vi "Waves.vi"(2 "Camera Queue":refnum<queue>, 3 "Wave Queue":refnum<queue>) -> (0 "error IO":errorcluster)   [LabVIEW 2016]
uses:
  controls/ModeEnum.ctl
  controls/Microscope Settings.ctl
  controls/ColourCalibration.ctl
  controls/CameraControlTypeDef.ctl
  controls/Hardware.ctl
  controls/PinOut.ctl
  <vilib>/Waveform/WDTOps.llb/WDT Waveform Duration DBL.vi
  <vilib>/DAQmx/create/channels.llb/DAQmx Create Channel (DO-Digital Output).vi
  <vilib>/DAQmx/create/channels.llb/DAQmx Create Channel (AO-Voltage-Basic).vi
panel:
  out "Duration":string
  out "Mixed Signal Graph 2":cluster{waveform(dbl)[], digitalwaveform[]}(graph)
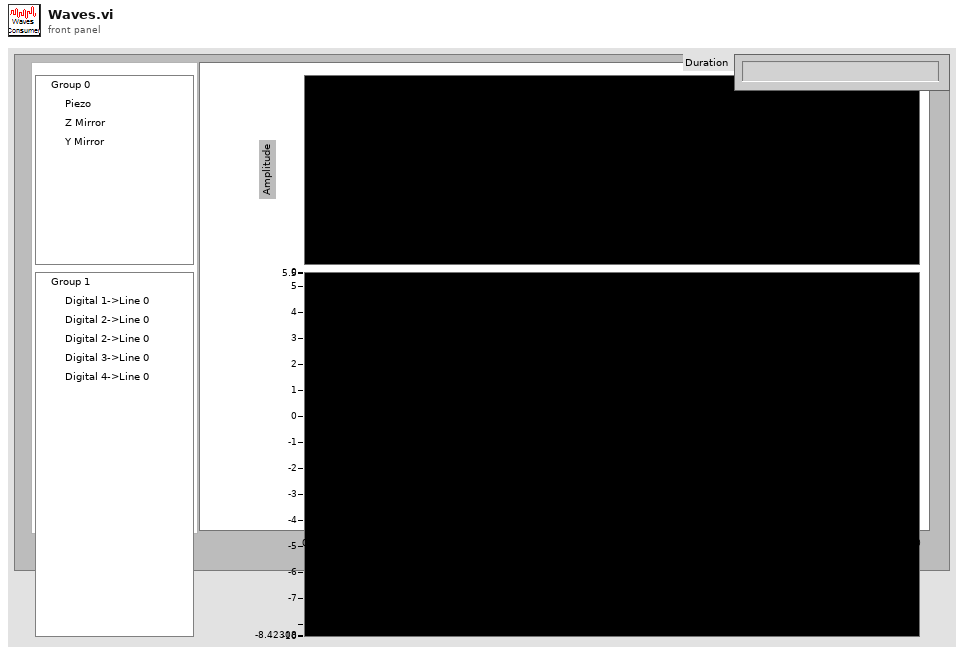
[diagram p1: front panel]
types:
  T1 = typedef "Microscope Settings.ctl" = cluster{"Mode":enum16{"Brightfield", "X", "XY", "XYZ", "XYZT", "XYZC", "Tweezers", "Virus"}, "Slit":cluster{"Scanning Mode":dbl, "Slit Width /%":dbl}, "Colour":T2, "Exposure/ms":dbl, "Piezo Position /um":dbl, "ROI":cluster{"X":cluster{"Start /px":dbl, "Step /px":dbl, "Range /px":dbl}, "Y":cluster{"Start /px":dbl, "Step /px":dbl, "Range /px":dbl}, "Z ":cluster{"Start /um":dbl, "Step/um":dbl, "Range /um":dbl}, "T ":cluster{"Start /s":dbl, "Step /s":dbl, "Range /s":dbl}}, "Samples per millisecond":dbl, "Relax/ms":dbl, "Readout Direction":dbl, "Trigger Source":dbl, "Camera Delay /ms":dbl, "Under Scan /ms":dbl, "Waveforms":cluster{"Analogue Out":waveform(dbl)[], "Digital Out":digitalwaveform[]}}
  T2 = typedef "ColourCalibration.ctl" = cluster{"Colour":cluster{"Laser":enum16{"Brightfield", "445", "488", "561", "647"}, "Filter":u16}, "Calibration Coordinates":cluster{"Top Left":dbl[], "Top Right":dbl[], "Bottom Left":dbl[], "Bottom Right":dbl[]}}[]
  T3 = typedef "Hardware.ctl" = enum16{"Stop", "RunCont", "EndCont", "Idle", "Update", "Run Waves"}
  T4 = typedef "ModeEnum.ctl" = enum16{"Idle", "Init", "generateWaves", "runWaves", "runWavesCont", "endWavesCont", "stop"}
  T5 = typedef "Microscope Settings.ctl" = cluster{"Mode":enum16{"Brightfield", "X", "XY", "XYZ", "XYZT", "XYZC", "Tweezers", "Virus"}, "Slit":cluster{"Scanning Mode":dbl, "Slit Width /%":dbl}, "Colour":cluster{"Laser":enum16{"Brightfield", "445", "488", "561", "647"}, "Filter":u16}[], "Exposure/ms":dbl, "Piezo Position /um":dbl, "ROI":cluster{"X":cluster{"Start /px":dbl, "Step /px":dbl, "Range /px":dbl}, "Y":cluster{"Start /px":dbl, "Step /px":dbl, "Range /px":dbl}, "Z ":cluster{"Start /um":dbl, "Step/um":dbl, "Range /um":dbl}, "T ":cluster{"Start /s":dbl, "Step /s":dbl, "Range /s":dbl}}, "Samples per millisecond":dbl, "Relax/ms":dbl, "Readout Direction":dbl, "Trigger Source":dbl, "Camera Delay /ms":dbl, "Under Scan /ms":dbl, "Calibration Coordinates":cluster{"Top Left":dbl[], "Top Right":dbl[], "Bottom Left":dbl[], "Bottom Right":dbl[], "Waveforms":cluster{"Analogue Out":waveform(dbl)[], "Digital Out":digitalwaveform[]}}}
  T6 = typedef "CameraControlTypeDef.ctl" = enum16{"Idle", "Init", "Close", "IntervalLineInt", "Ram Record", "HardDisk Record", "Disengage Update", "Update", "ROI", "Binning", "Scan Mode", "Trigger Mode", "Readout Mode", "Readout Direction", "Preview", "ROIWindow", "Trigger Source"}
  T7 = cluster{"Analogue":refnum<k21>, "Digital":refnum<k21>}
  T8 = typedef "PinOut.ctl" = string
  T9 = enum16{"Brightfield", "X", "XY", "XYZ", "XYZT", "XYZC", "Tweezers", "Virus"}
  T10 = cluster{"Start /um":dbl, "Step/um":dbl, "Range /um":dbl}
  T11 = cluster{"Analogue Out out":waveform(dbl)[], "Digital Out out":digitalwaveform[]}
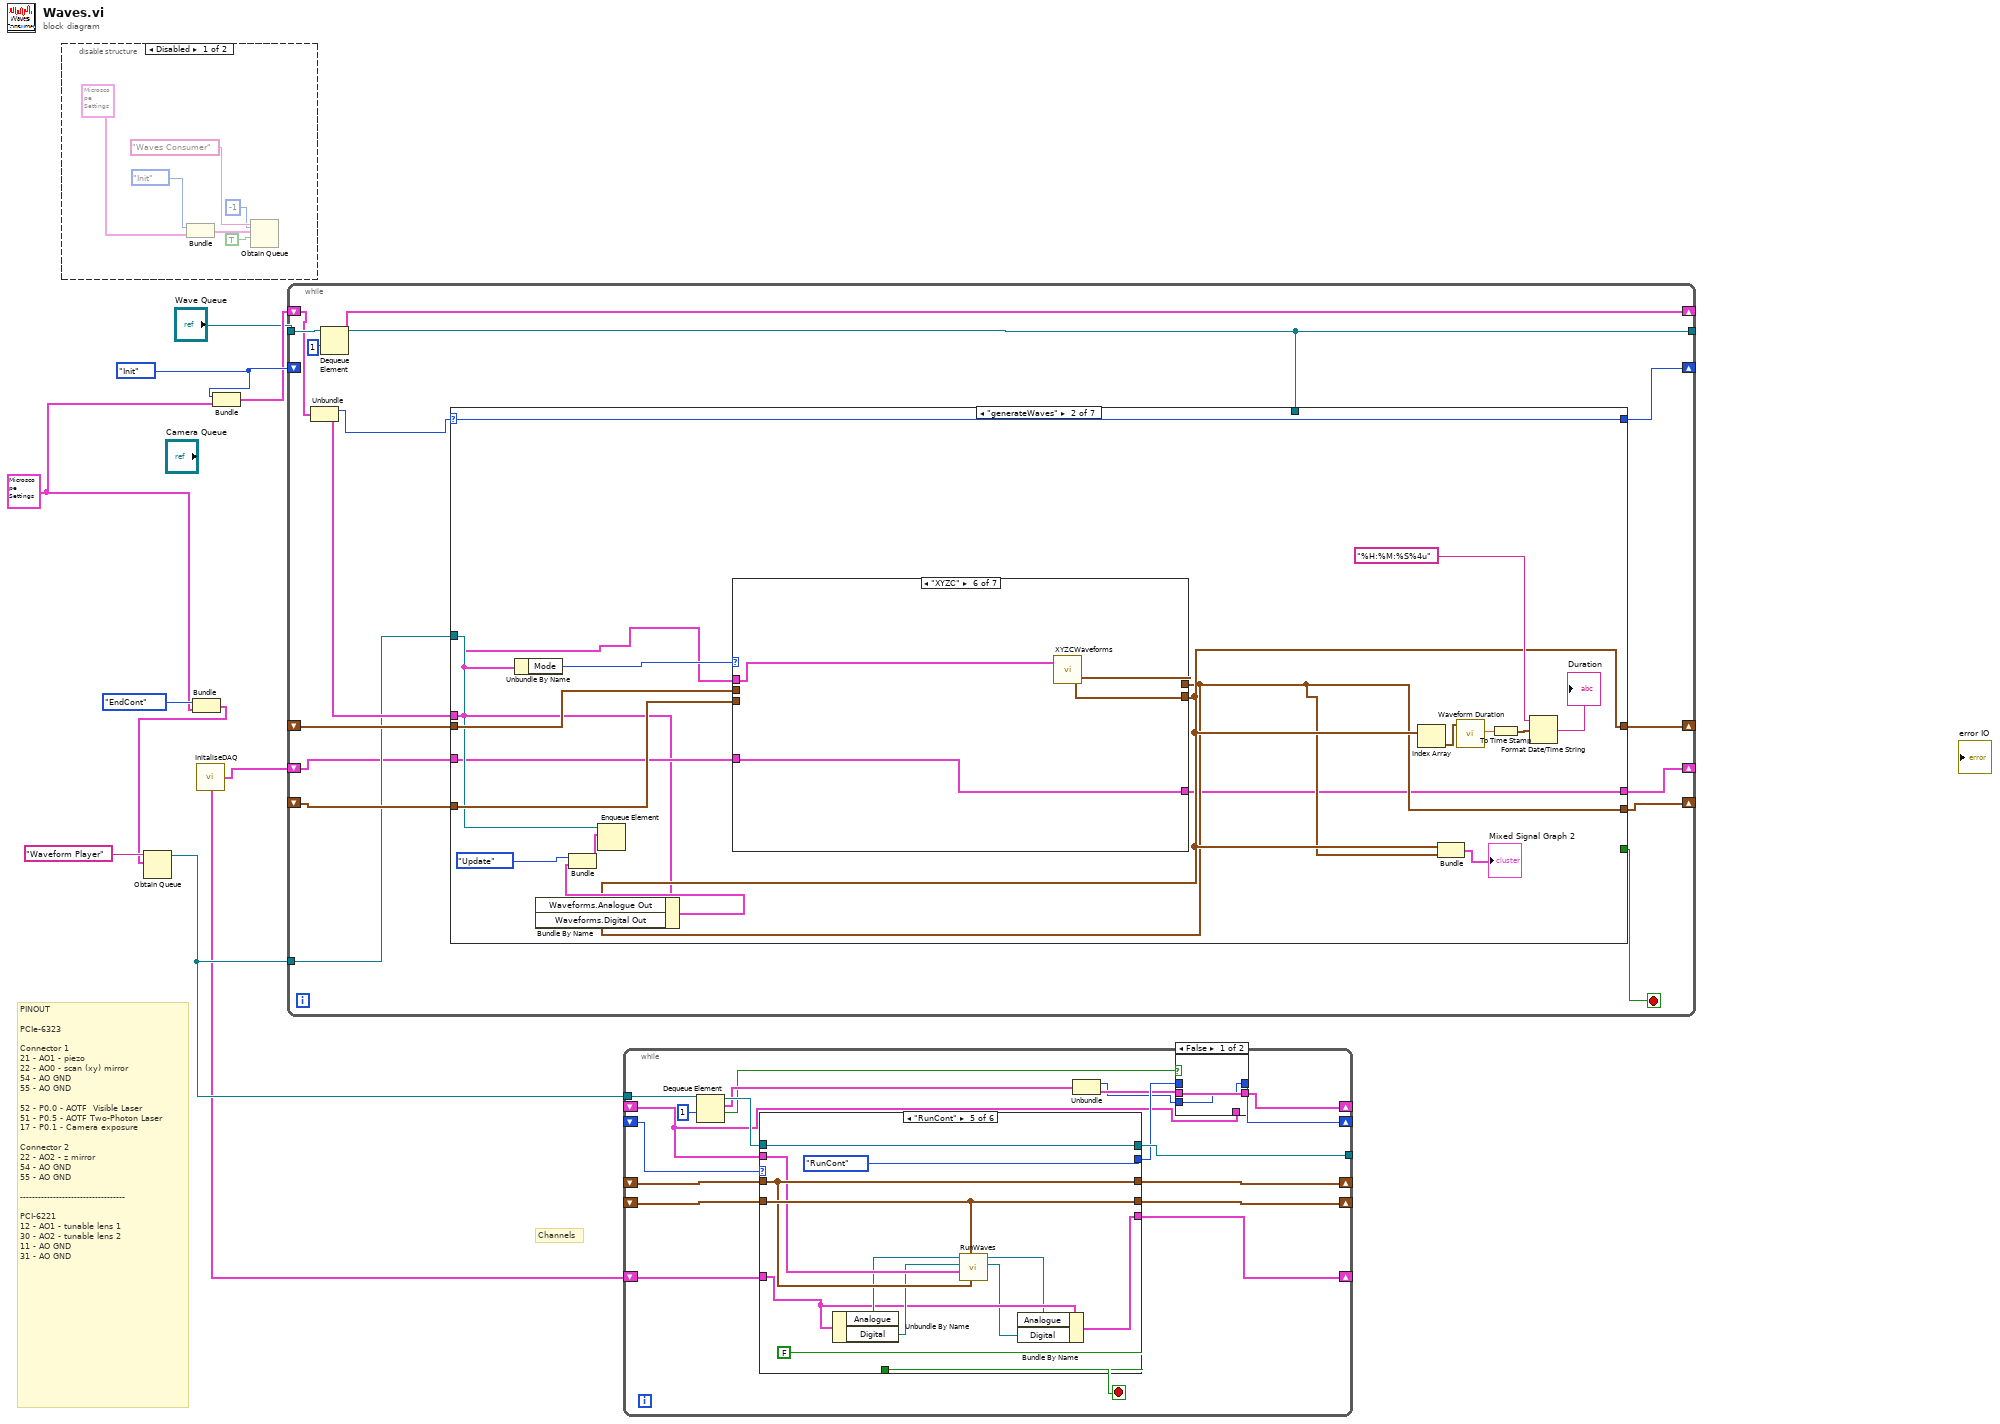
[diagram p0: block diagram]
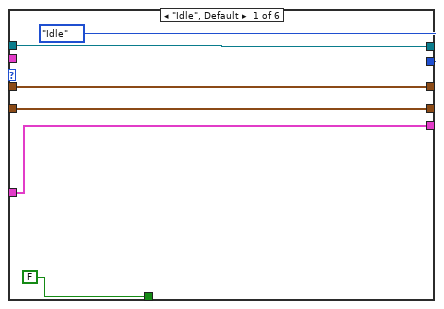
[diagram p3: hidden frame]
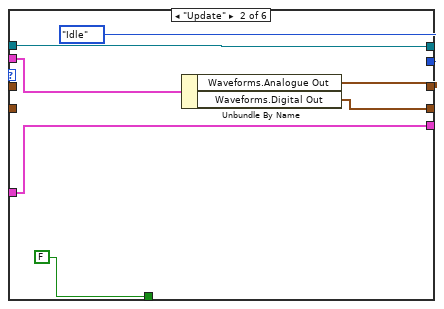
[diagram p4: hidden frame]
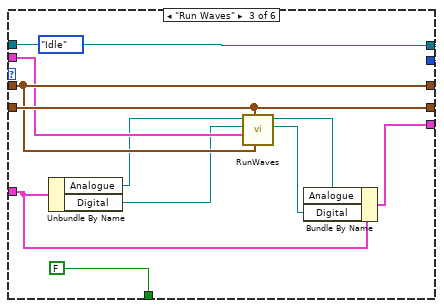
[diagram p5: hidden frame]
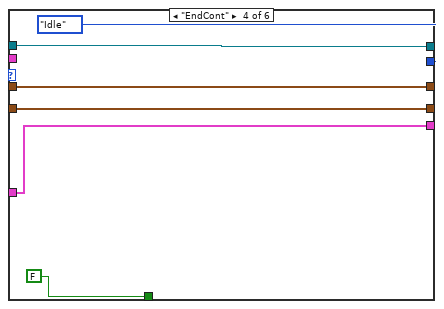
[diagram p6: hidden frame]
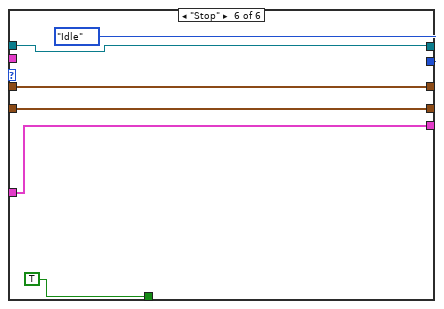
[diagram p7: hidden frame]
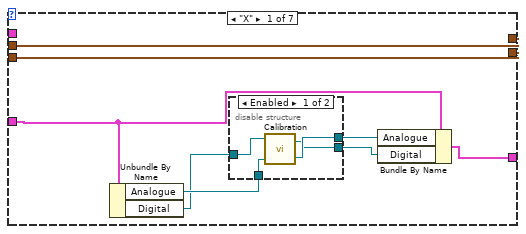
[diagram p9: hidden frame]
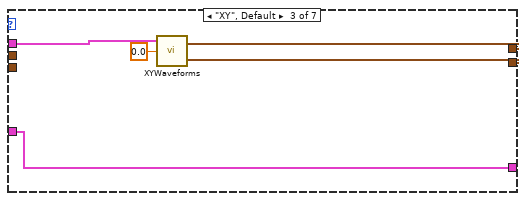
[diagram p12: hidden frame]
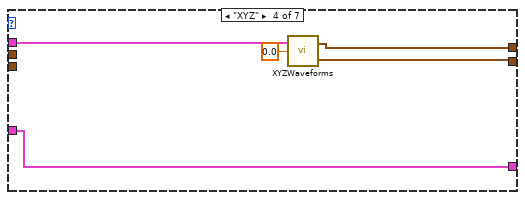
[diagram p13: hidden frame]
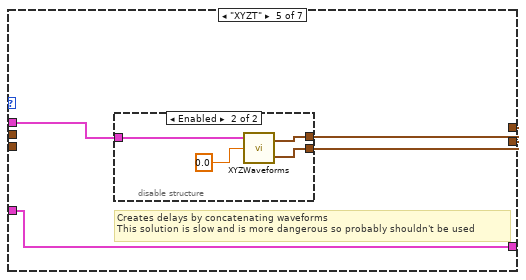
[diagram p14: hidden frame]
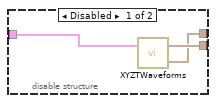
[diagram p15: hidden frame]
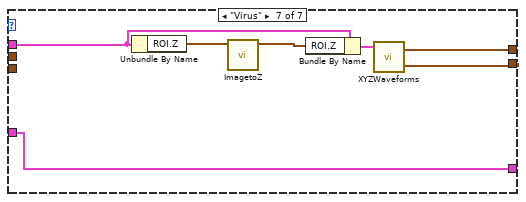
[diagram p16: hidden frame]
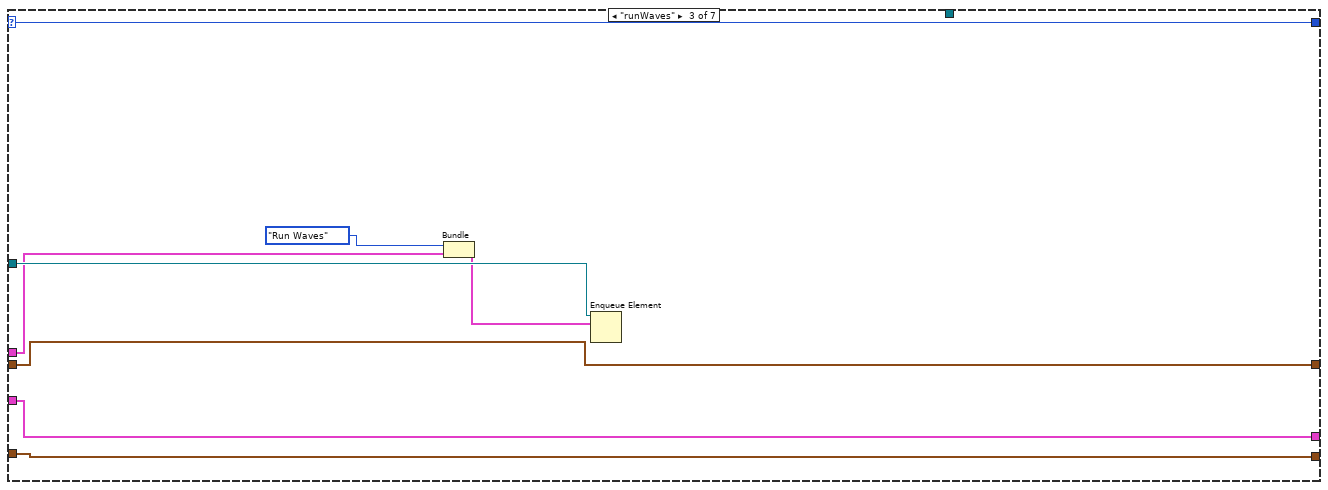
[diagram p17: hidden frame]
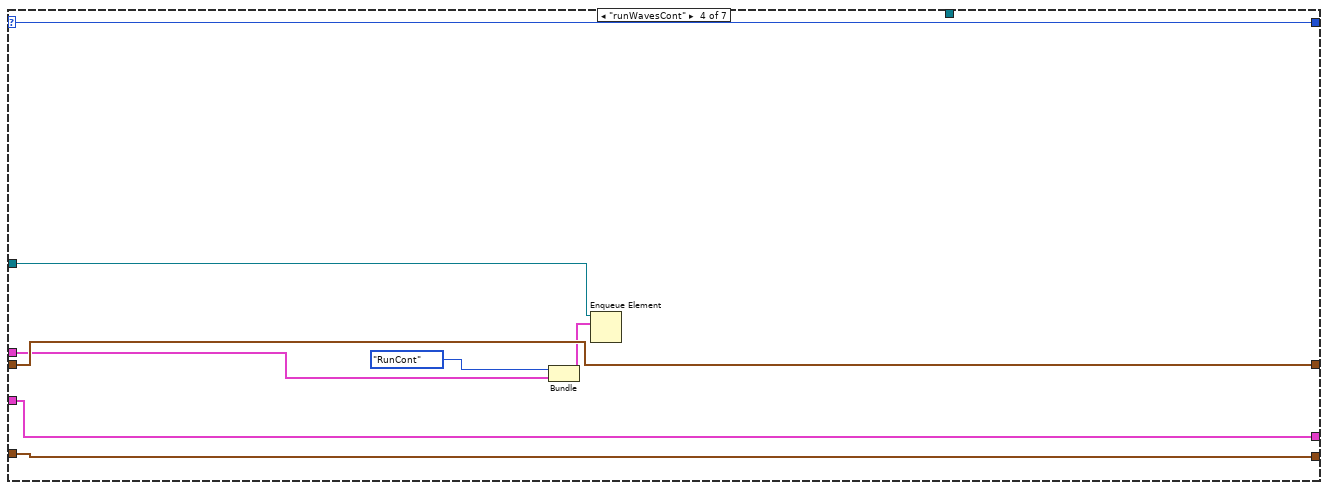
[diagram p18: hidden frame]
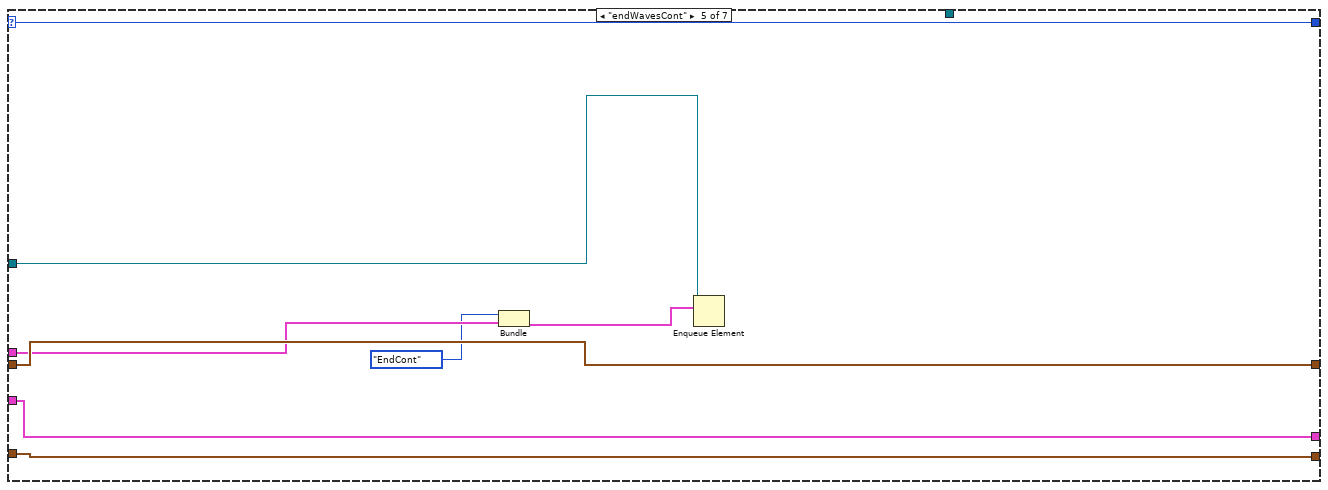
[diagram p19: hidden frame]
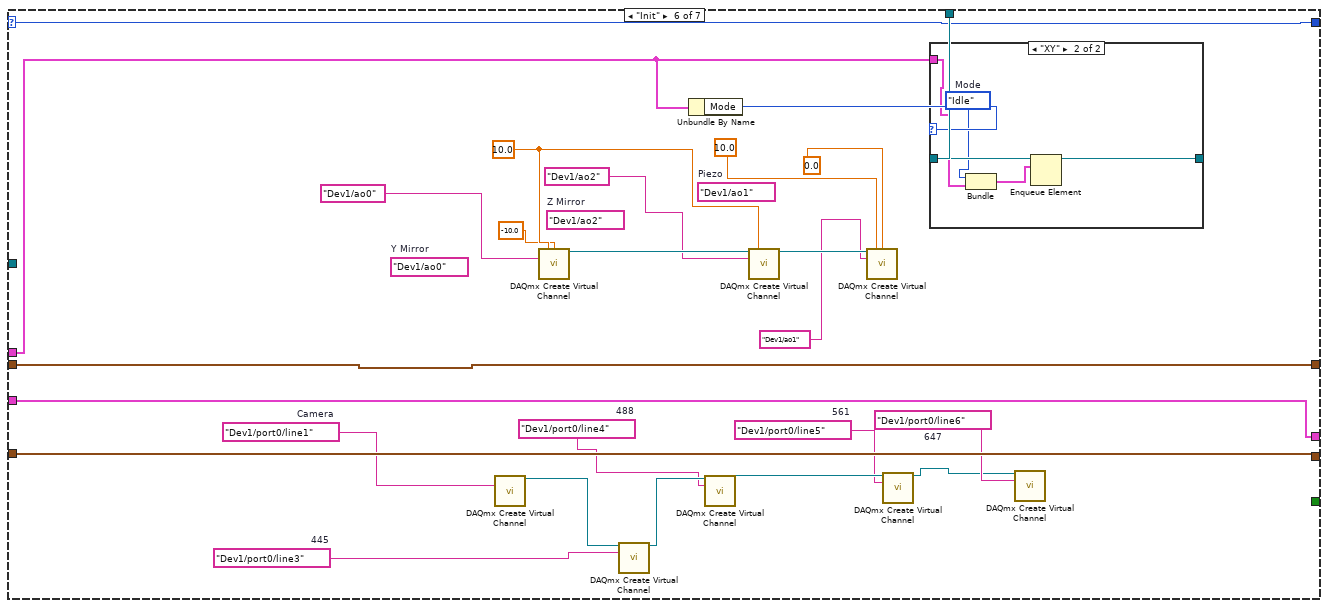
[diagram p20: hidden frame]
diagram:
  w1 = T1 {"Mode"=enum."XY", "Slit"={"Scanning Mode"=12.0, "Slit Width /%"=5.0}, "Colour"=[{"Colour"={"Laser"=enum."561", "Filter"=4}, "Calibration Coordinates"={"Top Left"=[-4.418670520231216, -0.1592138728323702, 10.0], "Top Right"=[-9.501965317919073, -0.1592138728323702, 10.0], "Bottom Left"=[-4.4508670520231215, 0.0, 0.0], "Bottom Right"=[-9.53757225433526, 0.0, 0.0]}}], "Exposure/ms"=40.0, "Piezo Position /um"=0.0, "ROI"={"X"={"Start /px"=0.0, "Step /px"=1.0, "Range /px"=2048.0}, "Y"={"Start /px"=0.0, "Step /px"=1.0, "Range /px"=2048.0}, "Z "={"Start /um"=0.0, "Step/um"=1.0, "Range /um"=100.0}, "T "={"Start /s"=0.0, "Step /s"=1.0, "Range /s"=100.0}}, "Samples per millisecond"=100.0, "Relax/ms"=10.0, "Readout Direction"=2.0, "Trigger Source"=2.0, "Camera Delay /ms"=11.0, "Under Scan /ms"=5.0, "Waveforms"={"Analogue Out"=[{"t0"=timestamp(0 s since 1904-01-01), "dt"=1.0, "Y"=[]}, {"t0"=timestamp(0 s since 1904-01-01), "dt"=1.0, "Y"=[]}, {"t0"=timestamp(0 s since 1904-01-01), "dt"=1.0, "Y"=[]}], "Digital Out"=[{"t0"=timestamp(0 s since 1904-01-01), "dt"=0.0, "Y"={"transitions"=[], "data"=[]}}, {"t0"=timestamp(0 s since 1904-01-01), "dt"=0.0, "Y"={"transitions"=[], "data"=[]}}, {"t0"=timestamp(0 s since 1904-01-01), "dt"=0.0, "Y"={"transitions"=[], "data"=[]}}]}} ("Microscope Settings")
  w7 = ModeEnum."Init" ("Mode")
  # "Channels"
  # "PINOUT\n\nPCIe-6323\n\nConnector 1\n21 - AO1 - piezo\n22 - AO0 - scan (xy) mirror\n54 - AO GND\n55 - AO GND\n\n52 - P0.0 - AOTF  Visible Laser\n51 - P0.5 - AOTF Two-Photon Laser\n17 - P0.1 - Camera exposure\n\nConnector 2\n22 - AO2 - z mirror\n54 - AO GND\n55 - AO GND\n\n-----------------------------------\n\nPCI-6221\n12 - AO1 - tunable lens 1\n30 - AO2 - tunable lens 2\n11 - AO GND\n31 - AO GND"
  n1 = disable-structure shown="Disabled" {
    frame Disabled {
      n2 = Bundle("Enum"=CameraControlTypeDef."Init", "Microscope Settings"=T5 {"Mode"=enum."X", "Slit"={"Scanning Mode"=12.0, "Slit Width /%"=5.0}, "Colour"=[{"Laser"=enum."561", "Filter"=4}], "Exposure/ms"=40.0, "Piezo Position /um"=0.0, "ROI"={"X"={"Start /px"=0.0, "Step /px"=1.0, "Range /px"=2048.0}, "Y"={"Start /px"=0.0, "Step /px"=1.0, "Range /px"=2048.0}, "Z "={"Start /um"=0.0, "Step/um"=1.0, "Range /um"=100.0}, "T "={"Start /s"=0.0, "Step /s"=1.0, "Range /s"=100.0}}, "Samples per millisecond"=100.0, "Relax/ms"=10.0, "Readout Direction"=2.0, "Trigger Source"=2.0, "Camera Delay /ms"=11.0, "Under Scan /ms"=5.0, "Calibration Coordinates"={"Top Left"=[-4.418670520231216, -0.1592138728323702, 10.0], "Top Right"=[-9.501965317919073, -0.1592138728323702, 10.0], "Bottom Left"=[-4.4508670520231215, 0.0, 0.0], "Bottom Right"=[-9.53757225433526, 0.0, 0.0], "Waveforms"={"Analogue Out"=[], "Digital Out"=[]}}}) -> (w12:cluster{"Enum":T6, "Microscope Settings":T5})  [unwired: 1 in]
      n3 = Obtain Queue(max queue size (-1, unlimited)=-1, name (unnamed)="Waves Consumer", element data type=w12, create if not found? (T)=TRUE) -> ()  [unwired: 1 in, 3 out]
    }
    frame Enabled {
    }
  }
  n4 = Bundle(Hardware."EndCont", "Microscope Settings"=w1) -> (w4:cluster{T3, "Microscope Settings":T1})  [unwired: 1 in]
  n5 = Obtain Queue(name (unnamed)="Waveform Player", element data type=w4) -> (queue out=w8:refnum<queue>)  [unwired: 3 in, 2 out]
  n6 = call "InitaliseDAQ.vi"() -> ("Channels"=w2:T7)
  n7 = Bundle("Mode"=w7, "Microscope Settings"=w1) -> (w5:cluster{"Mode":T4, "Microscope Settings":T1})  [unwired: 1 in]
  n8 = while {
    shift-right: [w19] -> _
    shift-left: w7 -> [_]
    tunnel: "Wave Queue" -> [w30]
    tunnel: [w20] -> _
    shift-right: [w29] -> _
    shift-left: w5 -> [w28]
    shift-right: [w26] -> _
    shift-left: _ -> [w24]
    shift-right: [w27] -> _
    shift-left: _ -> [w25]
    tunnel: w8 -> [w21]
    shift-right: [w16] -> _
    shift-left: w2 -> [w17]
    stop <- w18 stop-if-true
    n9 = Unbundle(w28) -> ("Mode"=w23:T4, "Microscope Settings"=w22:T1)
    n10 = Dequeue Element(queue=w30, timeout in ms (-1)=1) -> (queue out=w20:refnum<queue>, element=w29:cluster{"Mode":T4, "Microscope Settings":T1})  [unwired: 1 in, 2 out]
    n11 = case shown="\"generateWaves\"" w23 {
      selector: w23 -> [w33 w47 w109 w117 w125 w127 w162]
      tunnel: [_ _ _ _ _ _ TRUE] -> w18
      tunnel: w22 -> [_ w36 w105 w113 w121 w129 w159]
      tunnel: [w35 w41 w107 w115 w123 w150 w165] -> w27
      tunnel: w25 -> [w35 w52 w107 w115 w123 w150 w165]
      tunnel: [w34 w40 w106 w114 w122 w149 w164] -> w26
      tunnel: w24 -> [w34 w54 w106 w114 w122 w149 w164]
      tunnel: [w33 w47 w109 w117 w125 w127 w162] -> w19
      tunnel: w21 -> [_ w45 w108 w116 w124 _ w161]
      tunnel: w20 -> [_ _ _ _ _ w130 _]
      tunnel: w17 -> [w32 w38 w102 w110 w118 w126 w157]
      tunnel: [w32 w37 w102 w110 w118 w126 w157] -> w16
      frame "Idle", Default {
      }
      frame "generateWaves" {
        n12 = Unbundle By Name(w36) -> ("Mode"=w53:T9)
        n13 = case shown="\"XYZC\"" w53 {
          tunnel: [w62 w69 w73 w78 w83 w94 w100] -> w41
          tunnel: w36 -> [_ _ w74 w79 w81 w92 w99]
          tunnel: [w61 w68 w72 w77 w82 w93 w101] -> w40
          tunnel: w54 -> [w61 w68 _ _ _ _ _]
          tunnel: w52 -> [w62 w69 _ _ _ _ _]
          tunnel: w38 -> [w58 w67 w71 w76 w80 w91 w95]
          tunnel: [w55 w67 w71 w76 w80 w91 w95] -> w37
          frame "X" {
            n14 = Unbundle By Name(w58) -> ("Analogue"=w60:refnum<k21>, "Digital"=w59:refnum<k21>)
            n15 = disable-structure shown="Enabled" {
              disable-tunnel: w59 -> [w66 _]
              disable-tunnel: w60 -> [w65 _]
              disable-tunnel: [w64 _] -> w57
              disable-tunnel: [w63 _] -> w56
              frame Enabled {
                n16 = call "Calibration.vi"("Analogue In"=w65, "Digital In"=w66) -> ("Analogue In Out"=w64:refnum<k21>, "Digital Out"=w63:refnum<k21>)  [unwired: 2 in]
              }
              frame Disabled {
              }
            }
            n17 = Bundle By Name(cluster=w58, "Analogue"=w57, "Digital"=w56) -> (w55:T7)
          }
          frame "Brightfield" {
          }
          frame "XY", Default {
            n18 = call "XYWaveforms.vi"("Colour Channel"=0.0, "Microscope Settings"=w74) -> ("Analogue Out"=w73:waveform(dbl)[], "Digital Out"=w72:digitalwaveform[])  [unwired: 1 out]
          }
          frame "XYZ" {
            n19 = call "XYZWaveforms.vi"("Colour Channel"=0.0, "Microscope Settings"=w79) -> ("Analogue Out out"=w78:waveform(dbl)[], "Digital Out out"=w77:digitalwaveform[])  [unwired: 1 in]
          }
          frame "XYZT" {
            # "Creates delays by concatenating waveforms\nThis solution is slow and is more dangerous so probably shouldn't be used"
            n20 = disable-structure shown="Enabled" {
              disable-tunnel: [w86 w88] -> w83
              disable-tunnel: [w85 w89] -> w82
              disable-tunnel: w81 -> [w84 w90]
              frame Disabled {
                n21 = call "XYZTWaveforms.vi"("Microscope Settings"=w84) -> ("Digital Out"=w85:digitalwaveform[], "Analogue Out"=w86:waveform(dbl)[])  [unwired: 1 in]
              }
              frame Enabled {
                n22 = call "XYZWaveforms.vi"("Colour Channel"=0.0, "Microscope Settings"=w90) -> ("Analogue Out out"=w88:waveform(dbl)[], "Digital Out out"=w89:digitalwaveform[])  [unwired: 1 in]
              }
            }
          }
          frame "XYZC" {
            n23 = call "XYZCWaveforms.vi"("Microscope Settings"=w92) -> ("Array"=w93:digitalwaveform[], "Analogue Out out"=w94:waveform(dbl)[])  [unwired: 1 in]
          }
          frame "Virus" {
            n24 = Unbundle By Name(w99) -> ("ROI.Z"=w97:T10)
            n25 = call "ImagetoZ.vi"("Z"=w97) -> ("ROI.Z"=w96:T10)  [unwired: 10 in]
            n26 = Bundle By Name(cluster=w99, "ROI.Z"=w96) -> (w98:T1)
            n27 = call "XYZWaveforms.vi"("Microscope Settings"=w98) -> ("Analogue Out out"=w100:waveform(dbl)[], "Digital Out out"=w101:digitalwaveform[])  [unwired: 2 in]
          }
        }
        n28 = Bundle By Name(cluster=w36, "Waveforms.Analogue Out"=w41, "Waveforms.Digital Out"=w40) -> (w46:T1)
        n29 = Bundle(Hardware."Update", "Microscope Settings"=w46) -> (w44:cluster{T3, "Microscope Settings":T1})  [unwired: 1 in]
        n30 = Enqueue Element(queue=w45, element=w44) -> ()  [unwired: 2 in, 3 out]
        n31 = Index Array(array=w41) -> (element=w51:waveform(dbl))  [unwired: 1 in]
        n32 = Bundle("Analogue Out out"=w41, "Digital Out out"=w40) -> (→"Mixed Signal Graph 2":T11)  [unwired: 1 in]
        n33 = call-poly <vilib>:"Waveform Duration.vi"("waveform in"=w51) -> ("duration"=w49:dbl)  [unwired: 8 in, 2 out]
        n34 = To Time Stamp(1:w49) -> (0:w50:timestamp)
        n35 = Format Date/Time String(time format string (%c)="%H:%M:%S%4u", seconds (now)=w50) -> (date/time string=→"Duration":string)  [unwired: 1 in]
      }
      frame "runWaves" {
        n36 = Bundle(Hardware."Run Waves", "Microscope Settings"=w105) -> (w104:cluster{T3, "Microscope Settings":T1})  [unwired: 1 in]
        n37 = Enqueue Element(queue=w108, element=w104) -> ()  [unwired: 2 in, 3 out]
      }
      frame "runWavesCont" {
        n38 = Bundle(Hardware."RunCont", "Microscope Settings"=w113) -> (w112:cluster{T3, "Microscope Settings":T1})  [unwired: 1 in]
        n39 = Enqueue Element(queue=w116, element=w112) -> ()  [unwired: 2 in, 3 out]
      }
      frame "endWavesCont" {
        n40 = Bundle(Hardware."EndCont", "Microscope Settings"=w121) -> (w119:cluster{T3, "Microscope Settings":T1})  [unwired: 1 in]
        n41 = Enqueue Element(queue=w124, element=w119) -> ()  [unwired: 2 in, 3 out]
      }
      frame "Init" {
        (unwired) tag "Dev1/ao1"  # Piezo
        (unwired) tag "Dev1/ao2"  # Z Mirror
        (unwired) tag "Dev1/ao0"  # Y Mirror
        w139 = 10.0 ("maximum value")
        w141 = tag "Dev1/port0/line6"  # 647
        w143 = tag "Dev1/port0/line5"  # 561
        w148 = tag "Dev1/port0/line3"  # 445
        w145 = tag "Dev1/port0/line4"  # 488
        w142 = tag "Dev1/port0/line1"  # Camera
        n42 = call-poly <vilib>:"DAQmx Create Virtual Channel.vi"("lines"=w142) -> ("task out"=w147:refnum<k21>)  [unwired: 13 in, 1 out]
        n43 = call-poly <vilib>:"DAQmx Create Virtual Channel.vi"("maximum value"=w139, "minimum value"=-10.0, "physical channels"=T8 "Dev1/ao0" ("Combo Box")) -> ("task out"=w135:refnum<k21>)  [unwired: 11 in, 1 out]
        n44 = call-poly <vilib>:"DAQmx Create Virtual Channel.vi"("task in"=w147, "lines"=w148) -> ("task out"=w146:refnum<k21>)  [unwired: 12 in, 1 out]
        n45 = Unbundle By Name(w129) -> ("Mode"=w128:T9)
        n46 = call-poly <vilib>:"DAQmx Create Virtual Channel.vi"("task in"=w146, "lines"=w145) -> ("task out"=w144:refnum<k21>)  [unwired: 12 in, 1 out]
        n47 = call-poly <vilib>:"DAQmx Create Virtual Channel.vi"("task in"=w135, "maximum value"=w139, "physical channels"=T8 "Dev1/ao2" ("Combo Box")) -> ("task out"=w134:refnum<k21>)  [unwired: 11 in, 1 out]
        n48 = call-poly <vilib>:"DAQmx Create Virtual Channel.vi"("task in"=w134, "maximum value"=10.0 ("minimum value"), "minimum value"=0.0 ("maximum value"), "physical channels"=T8 "Dev1/ao1" ("Combo Box")) -> ()  [unwired: 10 in, 2 out]
        n49 = call-poly <vilib>:"DAQmx Create Virtual Channel.vi"("task in"=w144, "lines"=w143) -> ("task out"=w140:refnum<k21>)  [unwired: 12 in, 1 out]
        n50 = case shown="\"XY\"" w128 {
          tunnel: w130 -> [w151 w156]
          tunnel: w129 -> [_ w154]
          tunnel: [w151 w152] -> _
          frame "X", Default {
          }
          frame "XY" {
            w153 = ModeEnum."Idle"  # Mode
            n51 = Bundle("Mode"=w153, "Microscope Settings"=w154) -> (w155:cluster{"Mode":T4, "Microscope Settings":T1})  [unwired: 1 in]
            n52 = Enqueue Element(queue=w156, element=w155) -> (queue out=w152:refnum<queue>)  [unwired: 2 in, 2 out]
          }
        }
        n53 = call-poly <vilib>:"DAQmx Create Virtual Channel.vi"("task in"=w140, "lines"=w141) -> ()  [unwired: 12 in, 2 out]
      }
      frame "stop" {
        n54 = Bundle(Hardware."Stop", "Microscope Settings"=w159) -> (w158:cluster{T3, "Microscope Settings":T1})  [unwired: 1 in]
        n55 = Enqueue Element(queue=w161, element=w158) -> ()  [unwired: 2 in, 3 out]
      }
    }
  }
  n56 = while {
    tunnel: [w185] -> _
    tunnel: w8 -> [w184]
    shift-right: [w181] -> _
    shift-left: _ -> [w179]
    shift-right: [w180] -> _
    shift-left: _ -> [w178]
    shift-right: [w174] -> _
    shift-left: _ -> [w176]
    shift-right: [w171] -> _
    shift-left: _ -> [w169]
    shift-right: [w166] -> _
    shift-left: w2 -> [w167]
    stop <- w168 stop-if-true
    n57 = Dequeue Element(queue=w184, timeout in ms (-1)=1) -> (queue out=w183:refnum<queue>, element=w182:cluster{T3, "Microscope Settings":T1}, timed out?=w175:bool)  [unwired: 1 in, 1 out]
    n58 = case shown="\"RunCont\"" w176 {
      tunnel: [w195 w202 w210 w217 w228 w236] -> w185
      tunnel: w183 -> [w195 w202 w210 w217 w228 w236]
      tunnel: w169 -> [_ w200 w212 _ w230 _]
      tunnel: [w194 w199 w213 w219 w231 w238] -> w181
      tunnel: [w193 w198 w214 w220 w232 w237] -> w180
      tunnel: w179 -> [w194 _ w213 w219 w231 w238]
      tunnel: w178 -> [w193 _ w214 w220 w232 w237]
      tunnel: [FALSE FALSE FALSE FALSE FALSE TRUE] -> w168
      tunnel: [Hardware."Idle" Hardware."Idle" Hardware."Idle" Hardware."Idle" Hardware."RunCont" Hardware."Idle"] -> w173
      tunnel: w167 -> [w190 w196 w206 w215 w224 w233]
      tunnel: [w190 w196 w203 w215 w221 w233] -> w166
      frame "Idle", Default {
      }
      frame "Update" {
        n59 = Unbundle By Name(w200) -> ("Waveforms.Analogue Out"=w199:waveform(dbl)[], "Waveforms.Digital Out"=w198:digitalwaveform[])
      }
      frame "Run Waves" {
        n60 = Unbundle By Name(w206) -> ("Analogue"=w208:refnum<k21>, "Digital"=w207:refnum<k21>)
        n61 = call "RunWaves.vi"("Analogue Out"=w213, "Digital Out"=w214, "Microscope Settings"=w212, "Digital In"=w207, "Analogue  in"=w208) -> ("Digital Out"=w204:refnum<k21>, "Analogue Out"=w205:refnum<k21>)  [unwired: 5 in]
        n62 = Bundle By Name(cluster=w206, "Analogue"=w205, "Digital"=w204) -> (w203:T7)
      }
      frame "EndCont" {
      }
      frame "RunCont" {
        n63 = Unbundle By Name(w224) -> ("Analogue"=w226:refnum<k21>, "Digital"=w225:refnum<k21>)
        n64 = call "RunWaves.vi"("Analogue Out"=w231, "Digital Out"=w232, "Microscope Settings"=w230, "Digital In"=w225, "Analogue  in"=w226) -> ("Digital Out"=w222:refnum<k21>, "Analogue Out"=w223:refnum<k21>)  [unwired: 5 in]
        n65 = Bundle By Name(cluster=w224, "Analogue"=w223, "Digital"=w222) -> (w221:T7)
      }
      frame "Stop" {
      }
    }
    n66 = Unbundle(w182) -> (w170:T3, "Microscope Settings"=w172:T1)
    n67 = case shown="False" w175 {
      tunnel: [w186 w189] -> w174
      tunnel: w173 -> [_ w189]
      tunnel: [w187 w188] -> w171
      tunnel: w172 -> [w187 _]
      tunnel: w170 -> [w186 _]
      tunnel: w169 -> [_ w188]
      frame False {
      }
      frame True {
      }
    }
  }
